vi "Bind.vi"(7 "path override":path, 8 "error in (no error)":errorcluster, 10 "addr_":string, 11 "s_":u64) -> (0 "error out":errorcluster, 3 "s_ out":u64)   [LabVIEW 2025, in "LibZMQ.lvlib"]
doc: "ZMQ_EXPORT int zmq_bind (void *s_, const char *addr_);\n\nCreates an endpoint"
uses:
  LibZMQ.lvlib
  errno.vi
  strerror.vi
  <vilib>/Utility/error.llb/Error Cluster From Error Code.vi
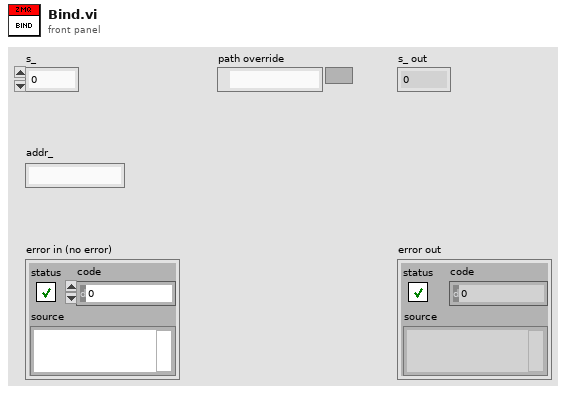
[diagram p1: front panel]
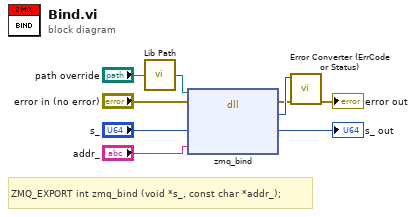
[diagram p0: block diagram]
diagram:
  # "ZMQ_EXPORT int zmq_bind (void *s_, const char *addr_);"
  n1 = call "Lib Path.vi"("path override"="path override") -> ("lib path"=w1:path)
  n2 = dll-call lib="home/james/Documents/ZeroMQ_LV/libzmq-v143-mt-4_3_6/libzmq.so" fn="zmq_bind"(path in=w1, error in="error in (no error)", "s_"="s_", "addr_"="addr_") -> (error out=w4:errorcluster, "return type"=w9:i32, "s_"=→"s_ out":u64)  [unwired: 2 in, 1 out]
  n3 = call "Error Converter (ErrCode or Status).vi"("error in (no error)"=w4, "error code"=w9) -> ("error out"=→"error out":errorcluster)  [unwired: 9 in]
